vi "populate_settings_combo.vi"(6 "force default settings":bool, 7 "default settings name":string, 8 "error in (no error)":errorcluster, 9 "available settings":T1[](array[typedef]), 10 "combo ref":refnum<vi>, 11 "ScanModeDL090923Scaffold in":refnum<class "ScanModeDL090923Scaffold.lvclass">=refnum) -> (0 "error out":errorcluster, 3 "ScanModeDL090923Scaffold out":refnum<class "ScanModeDL090923Scaffold.lvclass">)   [LabVIEW 2010]
uses:
  common/clusters/settings_specification_cluster.ctl
  ScanModeDL090923Scaffold.lvclass
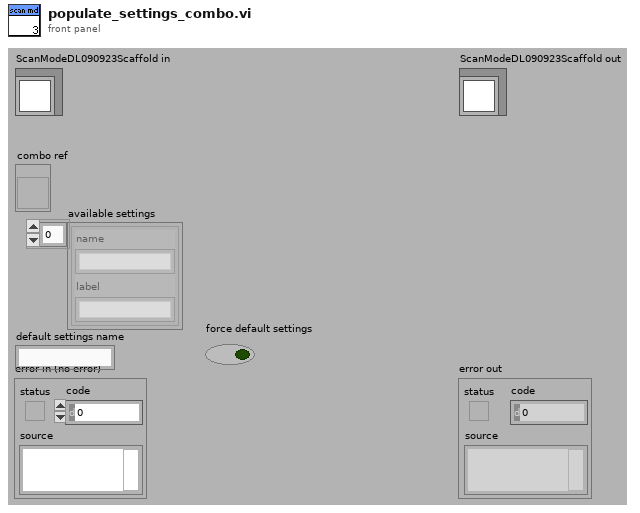
[diagram p1: front panel]
types:
  T1 = typedef "settings_specification_cluster.ctl" = cluster{"name":string, "label":string}
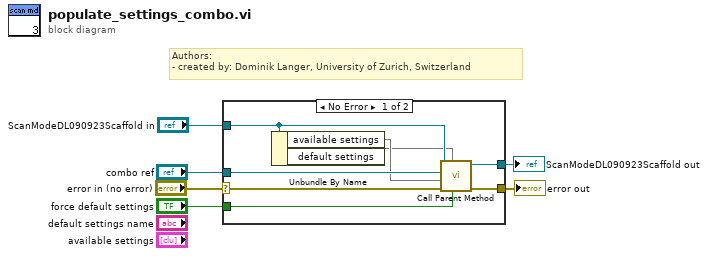
[diagram p0: block diagram]
diagram:
  # "Authors: \n- created by: Dominik Langer, University of Zurich, Switzerland"
  n1 = case shown="No Error" "error in (no error)" {
    selector: "error in (no error)" -> [w11 w15]
    tunnel: [w14 w15] -> w6
    tunnel: [w13 w16] -> w5
    tunnel: "combo ref" -> [w12 _]
    tunnel: "ScanModeDL090923Scaffold in" -> [w10 w16]
    tunnel: "force default settings" -> [w7 _]
    frame No Error {
      n2 = Unbundle By Name(w10) -> ("available settings"=w9, "default settings"=w8)
      n3 = call-parent "Call Parent Method"("force default settings"=w7, "default settings name"=w8, "error in (no error)"=w11, "combobox entries"=w9, "combo box ref"=w12, "GenericPlugin in"=w10) -> ("error out"=w14:errorcluster, "GenericPlugin out"=w13:refnum<class "ScanModeDL090923Scaffold.lvclass">)  [unwired: 4 in]
    }
    frame Error {
    }
  }
  "error out" <- w6
  "ScanModeDL090923Scaffold out" <- w5
